vi "grSim_Commands Encoder.vi"(8 "error in (no error)":errorcluster, 9 "Is Team Yellow?":bool=TRUE, 10 "robots":T1[](array[typedef]), 11 "Communication in":refnum<class "Communication.lvclass">) -> (0 "error out":errorcluster, 2 "robotControl":u8[](array[numeric]), 3 "Communication out":refnum<class "Communication.lvclass">)   [LabVIEW 2022 SP3, in "Communication.lvclass"]
uses:
  Communication.lvclass
  Paths/Convert AI Robot to Robot Command Folder/grSim/grSim Robot Command.ctl
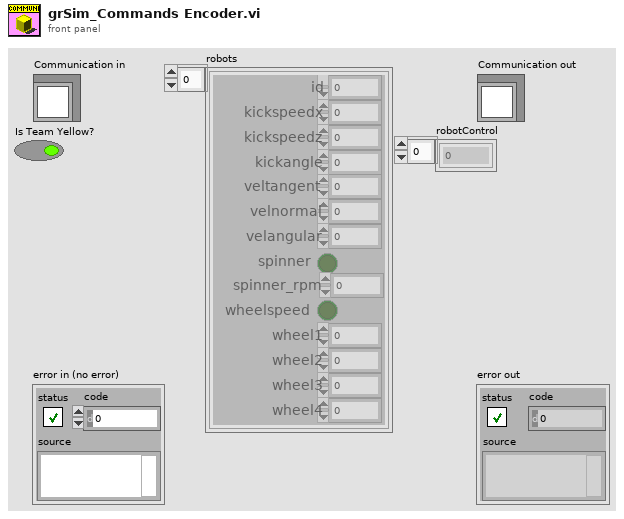
[diagram p1: front panel]
types:
  T1 = typedef "grSim Robot Command.ctl" = cluster{"id":u32, "kickspeedx":sgl, "kickspeedz":sgl, "veltangent":sgl, "velnormal":sgl, "velangular":sgl, "spinner":bool, "wheelspeed":bool, "wheel1":sgl, "wheel2":sgl, "wheel3":sgl, "wheel4":sgl, "kickangle":sgl, "spinner_rpm":sgl}
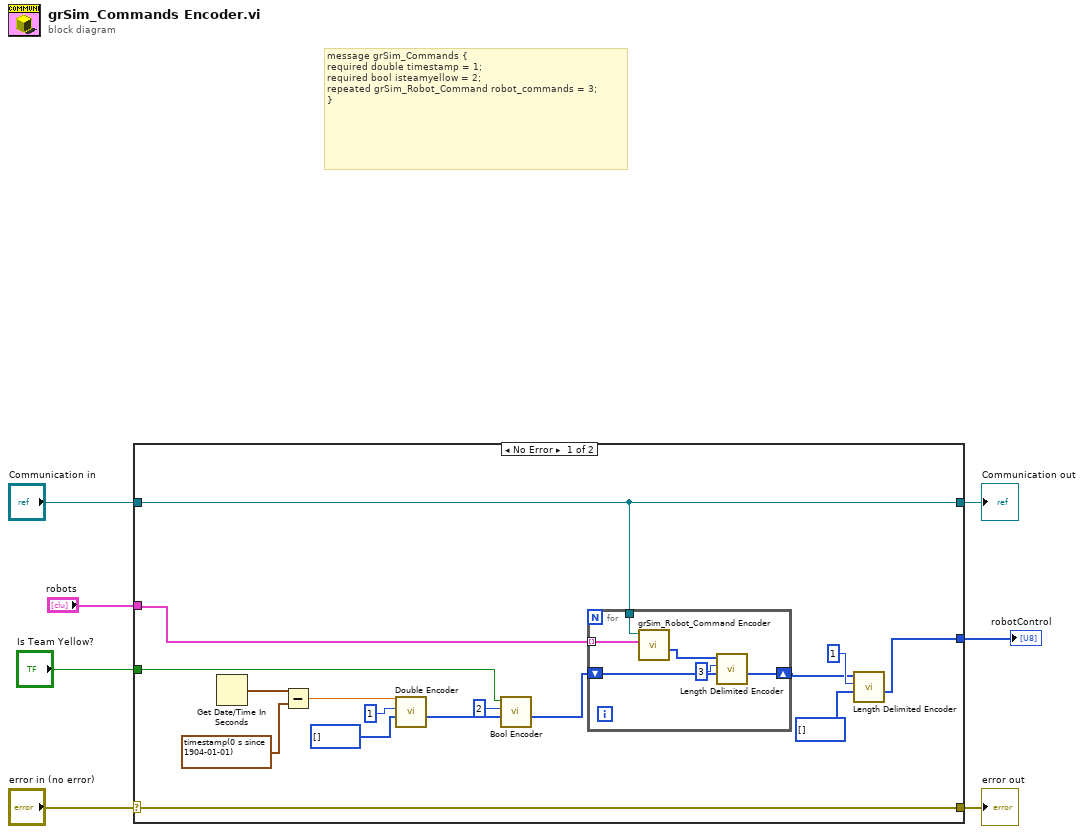
[diagram p0: block diagram]
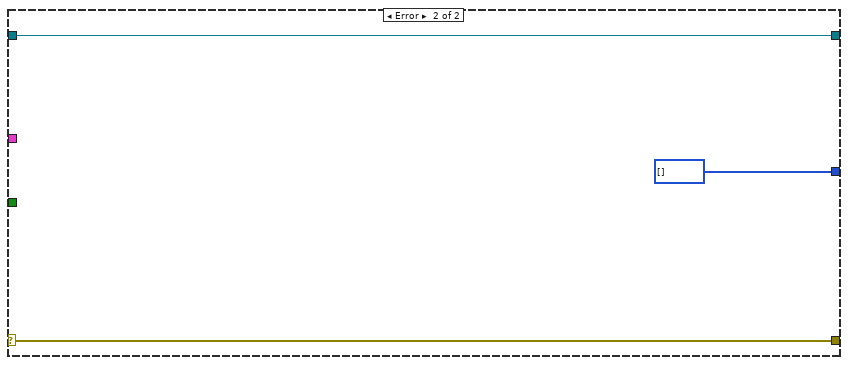
[diagram p2: hidden frame]
diagram:
  # "message grSim_Commands {\nrequired double timestamp = 1;\nrequired bool isteamyellow = 2;\nrepeated grSim_Robot_Command robot_commands = 3;\n}"
  n1 = case shown="No Error" "error in (no error)" {
    selector: "error in (no error)" -> [w23 w32]
    tunnel: [w23 w32] -> w6
    tunnel: [w14 w31] -> w4
    tunnel: "Communication in" -> [w14 w31]
    tunnel: "robots" -> [w9 _]
    tunnel: "Is Team Yellow?" -> [w8 _]
    tunnel: [w13 u8[] [] ("Array")] -> w1
    frame No Error {
      n2 = Get Date/Time In Seconds() -> (seconds since 1Jan1904=w22:timestamp)
      n3 = Subtract(x=w22, y=timestamp(0 s since 1904-01-01)) -> (x-y=w20:dbl)
      n4 = call "Double Encoder.vi"("Array In"=u8[] [] ("Array"), "Key"=u32 1, "Value"=w20) -> ("Array"=w17:u8[])  [unwired: 8 in]
      n5 = call "Bool Encoder.vi"("Array In"=w17, "Key"=u32 2, "Value"=w8) -> ("Array"=w15:u8[])  [unwired: 8 in]
      n6 = for {
        tunnel: w9 -> [w28] mode=indexing
        shift-right: [w25] -> w11
        shift-left: w15 -> [w27]
        tunnel: w14 -> [w24]
        n7 = call-dynamic "grSim_Robot_Command Encoder.vi"("robot"=w28, "Communication in"=w24) -> ("Array out"=w26:u8[])  [unwired: 7 in, 2 out]
        n8 = call "Length Delimited Encoder.vi"("Original Array In"=w27, "Key"=u32 3, "Array In to be added"=w26) -> ("Array"=w25:u8[])  [unwired: 8 in]
      }
      n9 = call "Length Delimited Encoder.vi"("Original Array In"=u8[] [] ("Array In to be added"), "Key"=u32 1, "Array In to be added"=w11) -> ("Array"=w13:u8[])  [unwired: 8 in]
    }
    frame Error {
    }
  }
  "error out" <- w6
  "Communication out" <- w4
  "robotControl" <- w1
